vi "StartData.vi"(8 "error in (no error)":errorcluster, 11 "RoomAlert In":refnum<class "RoomAlert.lvclass">) -> (0 "error out":errorcluster, 3 "RoomAlert Out":refnum<class "RoomAlert.lvclass">)   [LabVIEW 2018, in "SensorPlugins.lvlib" / "RoomAlert.lvclass"]
doc: "Starts the acquisition of measurements from the RoomAlert instrument."
uses:
  RoomAlert.lvclass
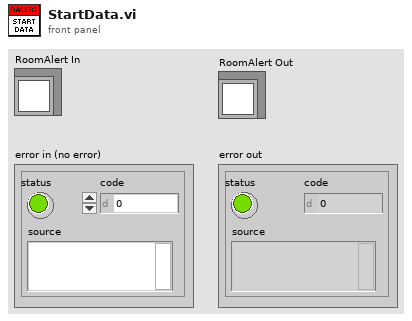
[diagram p1: front panel]
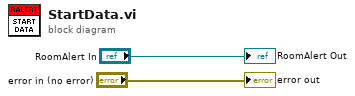
[diagram p0: block diagram]
diagram:
  "RoomAlert Out" <- "RoomAlert In"
  "error out" <- "error in (no error)"
